vi "Bitget 8-bits test.vi"(0 "x":i32) -> (20 "a":dbl, 21 "b":dbl, 22 "c":dbl, 23 "d":dbl, 24 "e":dbl, 25 "f":dbl, 26 "g":dbl, 27 "h":dbl)   [LabVIEW 2022 SP3]
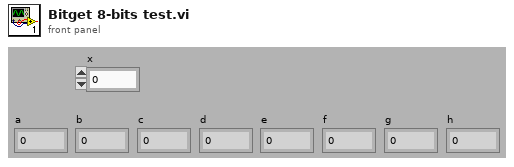
[diagram p1: front panel]
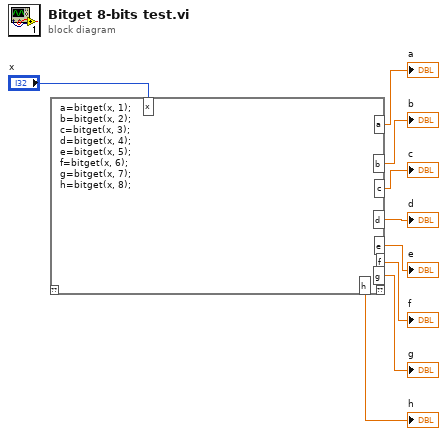
[diagram p0: block diagram]
diagram:
  n1 = script code="a=bitget(x, 1);\nb=bitget(x, 2);\nc=bitget(x, 3);\nd=bitget(x, 4);\ne=bitget(x, 5);\nf=bitget(x, 6);\ng=bitget(x, 7);\nh=bitget(x, 8);"("x"="x") -> ("a"=→"a":dbl, "b"=→"b":dbl, "c"=→"c":dbl, "d"=→"d":dbl, "e"=→"e":dbl, "f"=→"f":dbl, "g"=→"g":dbl, "h"=→"h":dbl)  [unwired: 1 in, 1 out]
